vi "CAN Interface Name Menu Item Count.vi"() -> (2 "number of menu items":u16)   [LabVIEW 2020, in "Communication Bus Template System Explorer.lvlib" / "Implementation.lvlib"]
uses:
  Implementation.lvlib
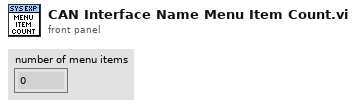
[diagram p1: front panel]
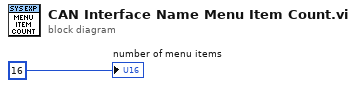
[diagram p0: block diagram]
diagram:
  "number of menu items" <- u16 16 ("number of menu items")
